vi "dfd_Remez Estimate N.vi"(6 "fs [Hz]":dbl=1.0 format="%.2f", 7 "auto order":bool, 8 "error in (no error)":errorcluster, 9 "band ripple":dbl[](array[numeric]) format="%.3e", 10 "band parameters":T1[](array[typedef])=[{"band specification"=[{"freq"=0.0, "amplitude"=1.0, "weight"=1.0}, {"freq"=0.2, "amplitude"=1.0, "weight"=1.0}], "ripple constraint"=0.0}, {"band specification"=[{"freq"=0.3, "amplitude"=0.0, "weight"=1.0}, {"freq"=0.5, "amplitude"=0.0, "weight"=1.0}], "ripple constraint"=0.0}]) -> (0 "error out":errorcluster, 2 "band parameters dup":T1[](array[typedef])=[{"band specification"=[{"freq"=0.0, "amplitude"=1.0, "weight"=1.0}, {"freq"=0.2, "amplitude"=1.0, "weight"=1.0}], "ripple constraint"=0.0}, {"band specification"=[{"freq"=0.3, "amplitude"=0.0, "weight"=1.0}, {"freq"=0.5, "amplitude"=0.0, "weight"=1.0}], "ripple constraint"=0.0}], 3 "estimated order":i32, 5 "minimum order":enum32{"user defined", "minEven", "minOdd"}(ring))   [LabVIEW 2017, in "NI_DigFilterLicensed.lvlib"]
uses:
  <vilib>/addons/Digital Filter Design/NI_DigFilterLicensed.lvlib
  <vilib>/addons/Digital Filter Design/_Objects.llb/DFD Adv Band Spec.ctl
  <vilib>/Analysis/baseanly.llb/Real A x B.vi
  <vilib>/Analysis/NI_AALBase.lvlib
panel:
  # "freq"
  # "amplitude"
  # "weight"
  # "freq"
  # "amplitude"
  # "weight"
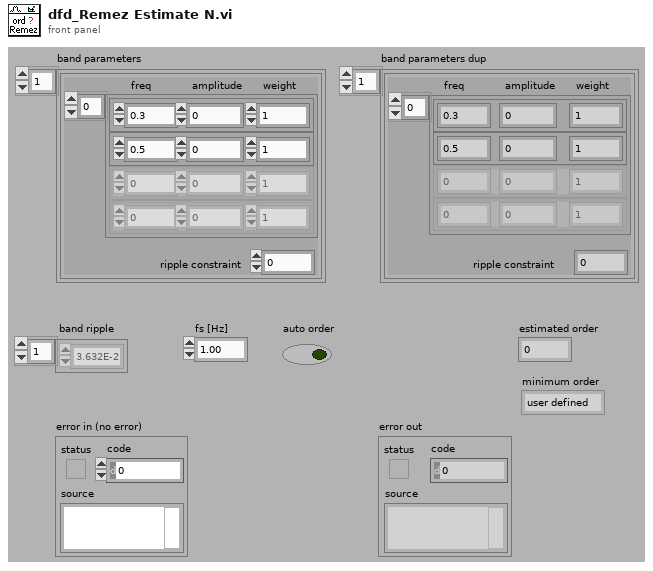
[diagram p1: front panel]
types:
  T1 = typedef "NI_DigFilterLicensed.lvlib/DFD Adv Band Spec.ctl" = cluster{"band specification":cluster{"freq":dbl, "amplitude":dbl, "weight":dbl}[], "ripple constraint":dbl}
  T2 = cluster{"freq":dbl, "amplitude":dbl, "weight":dbl}[]
  T3 = cluster{"freq":dbl, "amplitude":dbl, "weight":dbl}
  T4 = typedef "NI_Matrix.lvlib/RealMatrix.ctl" = dbl[][]
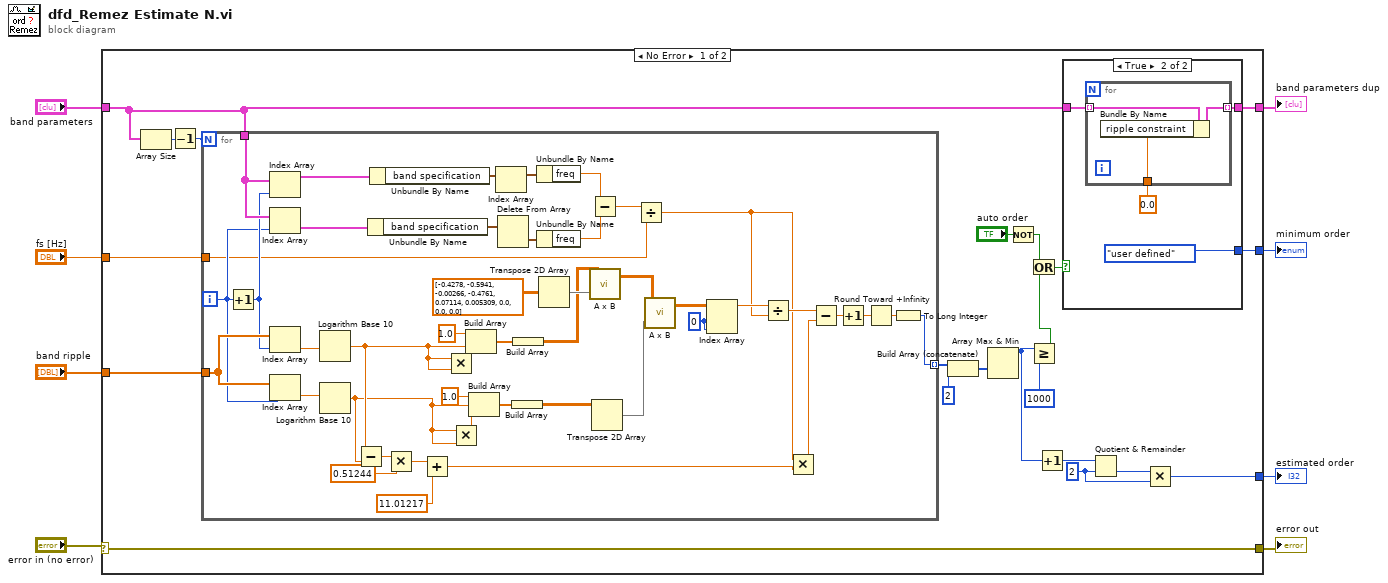
[diagram p0: block diagram]
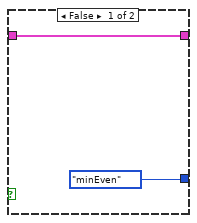
[diagram p2: hidden frame]
diagram:
  n1 = case shown="No Error" "error in (no error)" {
    selector: "error in (no error)" -> [w13 w84]
    tunnel: "fs [Hz]" -> [w26 _]
    tunnel: "band ripple" -> [w25 _]
    tunnel: [w11 _] -> w6
    tunnel: "band parameters" -> [w22 _]
    tunnel: [w21 _] -> w4
    tunnel: [w20 _] -> w3
    tunnel: [w13 w84] -> w1
    frame No Error {
      w9 = 2 ("y")
      n2 = Array Size(array=w22) -> (size(s)=w29:i32)
      n3 = Decrement(x=w29) -> (x-1=w28:i32)
      n4 = for {
        N: w28 -> [_]
        tunnel: w22 -> [w83]
        tunnel: [w80] -> w27 mode=indexing
        tunnel: w26 -> [w48]
        tunnel: w25 -> [w74]
        i -> [w72]
        w56 = 0 ("index (row)")
        n5 = Increment(x=w72) -> (x+1=w73:i32)
        n6 = Index Array(array=w83, index=w73) -> (element=w81:T1)
        n7 = Index Array(array=w83, index=w72) -> (element=w82:T1)
        n8 = Index Array(array=w74, index=w73) -> (element=w55:dbl)
        n9 = Index Array(array=w74, index=w72) -> (element=w54:dbl)
        n10 = Logarithm Base 10(1:w55) -> (0:w40:dbl)
        n11 = Logarithm Base 10(1:w54) -> (0:w39:dbl)
        n12 = Subtract(x=w40, y=w39) -> (x-y=w53:dbl)
        n13 = Unbundle By Name(w82) -> ("band specification"=w71:T2)
        n14 = Unbundle By Name(w81) -> ("band specification"=w79:T2)
        n15 = Multiply(x=w53, y=0.51244) -> (x*y=w51:dbl)
        n16 = Add(x=w51, y=11.01217) -> (x+y=w47:dbl)
        n17 = Multiply(x=w40, y=w40) -> (x*y=w66:dbl)
        n18 = Multiply(x=w39, y=w39) -> (x*y=w65:dbl)
        n19 = Build Array(1.0 ("element"), w40, w66) -> (w63:dbl[])
        n20 = Build Array(1.0 ("element"), w39, w65) -> (w60:dbl[])
        n21 = Index Array(array=w79) -> (element=w77:T3)  [unwired: 1 in]
        n22 = Delete From Array(array=w71) -> (deleted portion=w78:T3)  [unwired: 2 in, 1 out]
        n23 = Build Array(w60) -> (w59:dbl[][])
        n24 = Build Array(w63) -> (w62:dbl[][])
        n25 = Unbundle By Name(w77) -> ("freq"=w76:dbl)
        n26 = Unbundle By Name(w78) -> ("freq"=w75:dbl)
        n27 = Transpose 2D Array(2D array=dbl[][] [[-0.4278, -0.5941, -0.00266], [-0.4761, 0.07114, 0.005309], [0.0, 0.0, 0.0]] ("B")) -> (transposed array=w68:dbl[][])
        n28 = Subtract(x=w76, y=w75) -> (x-y=w49:dbl)
        n29 = call-poly <vilib>:"A x B.vi"("B"=w68, "A"=w62) -> ("A x B"=w61:T4)  [unwired: 1 out]
        n30 = Transpose 2D Array(2D array=w59) -> (transposed array=w58:dbl[][])
        n31 = Divide(x=w49, y=w48) -> (x/y=w41:dbl)
        n32 = call-poly <vilib>:"A x B.vi"("B"=w58, "A"=w61) -> ("A x B"=w57:T4)  [unwired: 1 out]
        n33 = Index Array(array=w57, index (row)=w56, index (col)=w56) -> (element=w46:dbl)
        n34 = Divide(x=w46, y=w41) -> (x/y=w45:dbl)
        n35 = Multiply(x=w41, y=w47) -> (x*y=w44:dbl)
        n36 = Subtract(x=w45, y=w44) -> (x-y=w43:dbl)
        n37 = Increment(x=w43) -> (x+1=w42:dbl)
        n38 = Round Toward +Infinity(x=w42) -> (ceil(x): smallest int >= x=w70:dbl)
        n39 = To Long Integer(number=w70) -> (32bit integer=w80:i32)
      }
      n40 = Build Array (concatenate)(w27, 2) -> (w15:i32[])
      n41 = Array Max & Min(array=w15) -> (max value=w24:i32)  [unwired: 3 out]
      n42 = Not(x="auto order") -> (.not. x?=w16:bool)
      n43 = Greater Or Equal?(x=w24, y=1000) -> (x >= y?=w18:bool)
      n44 = Or(x=w16, y=w18) -> (x .or. y?=w17:bool)
      n45 = Increment(x=w24) -> (x+1=w12:i32)
      n46 = case shown="True" w17 {
        tunnel: w22 -> [w31 w35]
        tunnel: [w31 w34] -> w21
        tunnel: [enum32{"user defined", "minEven", "minOdd"}."minEven" ("minimum order") enum32{"user defined", "minEven", "minOdd"}."user defined" ("minimum order")] -> w20
        frame False {
        }
        frame True {
          n47 = for {
            tunnel: w35 -> [w38] mode=indexing
            tunnel: [w37] -> w34 mode=indexing
            tunnel: 0.0 -> [w36]
            n48 = Bundle By Name(cluster=w38, "ripple constraint"=w36) -> (w37:T1)
          }
        }
      }
      n49 = Quotient & Remainder(x=w12, y=w9) -> (floor(x/y)=w10:i32)  [unwired: 1 out]
      n50 = Multiply(x=w10, y=w9) -> (x*y=w11:i32)
    }
    frame Error {
    }
  }
  "estimated order" <- w6
  "band parameters dup" <- w4
  "error out" <- w1
  "minimum order" <- w3
